vi "保存所有数据.vi"(6 "光强度":dbl, 8 "循环计数":dbl, 9 "移位输入":string[][](array[string]), 10 "湿度簇":T2, 11 "温度簇":T1) -> (3 "移位输出":string[][](array[string]))   [LabVIEW 2012]
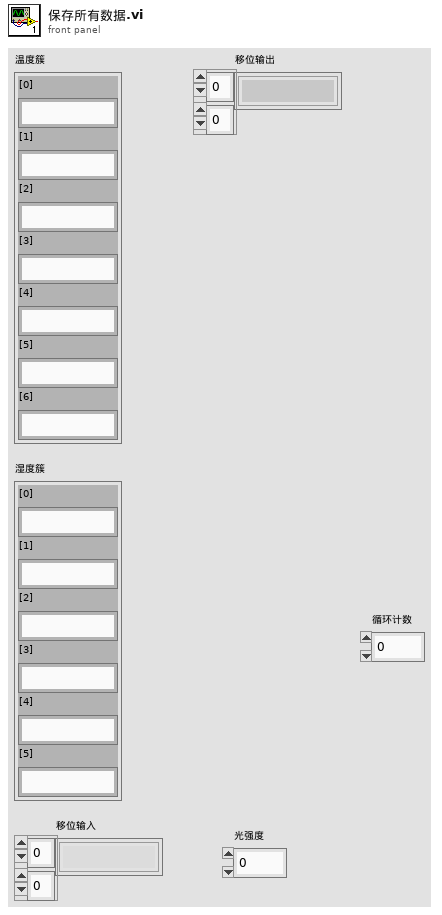
[diagram p1: front panel]
types:
  T1 = cluster{"[0]":string, "[1]":string, "[2]":string, "[3]":string, "[4]":string, "[5]":string, "[6]":string}
  T2 = cluster{"[0]":string, "[1]":string, "[2]":string, "[3]":string, "[4]":string, "[5]":string}
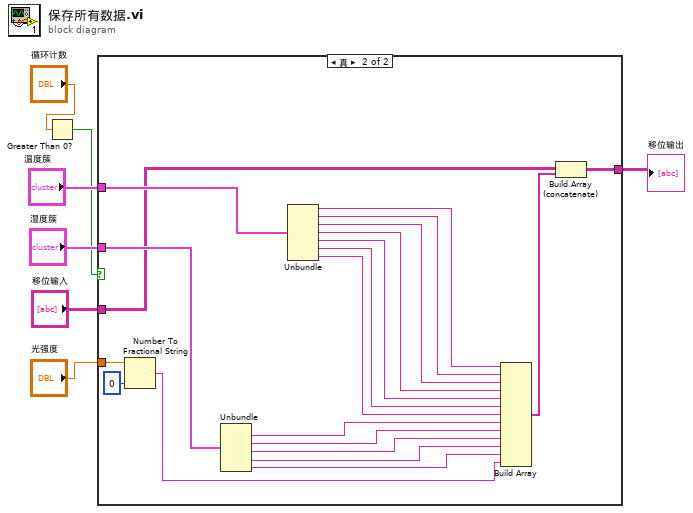
[diagram p0: block diagram]
diagram:
  n1 = Greater Than 0?(x="循环计数") -> (x > 0?=w2:bool)
  n2 = case shown="真" w2 {
    tunnel: [_ w27] -> w7
    tunnel: "湿度簇" -> [_ w25]
    tunnel: "温度簇" -> [_ w24]
    tunnel: "移位输入" -> [_ w23]
    tunnel: "光强度" -> [_ w10]
    frame False {
    }
    frame True {
      n3 = Number To Fractional String(number=w10, precision (6)=i16 0 ("精度(6)")) -> (F-format string=w9:string)  [unwired: 2 in]
      n4 = Unbundle(w25) -> ("[1]"=w16:string, "[2]"=w15:string, "[3]"=w14:string, "[4]"=w13:string, "[5]"=w12:string)  [unwired: 1 out]
      n5 = Unbundle(w24) -> ("[0]"=w22:string, "[1]"=w21:string, "[2]"=w20:string, "[3]"=w19:string, "[4]"=w18:string, "[5]"=w17:string, "[6]"=w11:string)
      n6 = Build Array(w22, w21, w20, w19, w18, w17, w11, w16, w15, w14, w13, w12, w9) -> (w26:string[])
      n7 = Build Array (concatenate)(w23, w26) -> (w27:string[][])
    }
  }
  "移位输出" <- w7
